vi "HH Cmd Interface.vi"(8 "error in":errorcluster, 9 "Device Inputs":dbl[](array[numeric]), 10 "DCM Ref":refnum<class "DCM - RT.lvclass">, 11 "HH in":T1) -> (0 "error out":errorcluster)   [LabVIEW 2016, in "DCM Engine.lvlib"]
uses:
  DCM Engine.lvlib
  Shared/Types/HH.ctl
  Shared/Types/HH Command Indexes.ctl
  Built/DCM Classes Packed/Pharlap/C/DCM-Classes.lvlibp/DCM/Rev0/RT/DCM - RT.lvclass
  Built/DCM Classes Packed/Pharlap/C/DCM-Classes.lvlibp/DCM/HH/RT/Setup.ctl
  Built/DCM Classes Packed/Pharlap/C/DCM-Classes.lvlibp/1abvi3w/vi.lib/Powertrain Controls/Device Drivers/DCM/HH/FPGA/Mode.ctl
  Built/DCM Classes Packed/Pharlap/C/DCM-Classes.lvlibp/1abvi3w/vi.lib/Powertrain Controls/Device Drivers/DCM/Rev0/FPGA/Digital Channel.ctl
  Built/DCM Classes Packed/Pharlap/C/DCM-Classes.lvlibp/DCM/HH/RT/Angle Control.ctl
  Built/DCM Classes Packed/Pharlap/C/DCM-Classes.lvlibp/DCM/HH/RT/DCM - RT - HH.lvlib
  Built/DCM Classes Packed/Pharlap/C/DCM-Classes.lvlibp/1abvi3w/vi.lib/Powertrain Controls/Device Drivers/DCM/HH/FPGA/DCM - FPGA - HH.lvlib
  Built/DCM Classes Packed/Pharlap/C/DCM-Classes.lvlibp/1abvi3w/vi.lib/Powertrain Controls/Device Drivers/DCM/Rev0/FPGA/DCM - FPGA.lvlib
  DCM Shared.lvlib
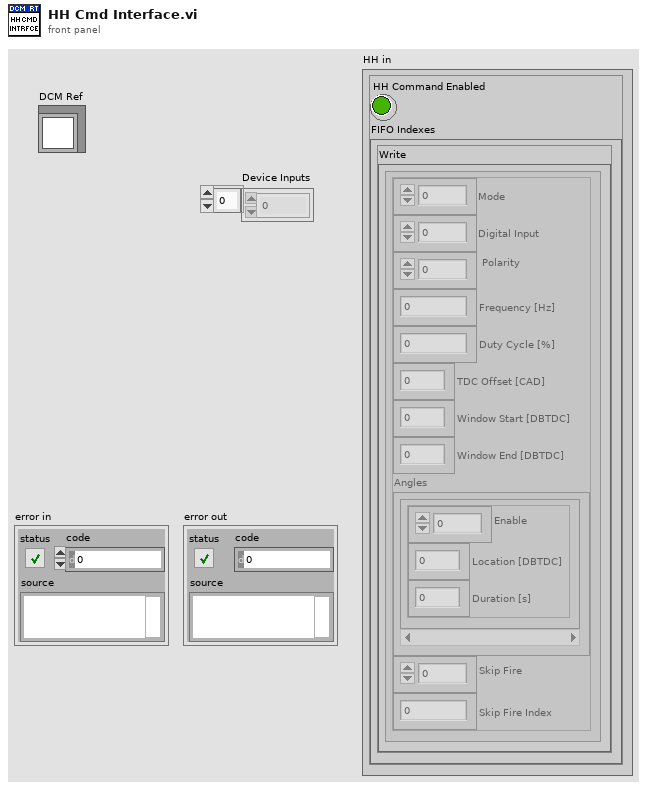
[diagram p1: front panel]
types:
  T1 = typedef "DCM Shared.lvlib/HH.ctl" = cluster{"HH Command Enabled":bool, "FIFO Indexes":cluster{"Write":T2[]}}
  T2 = typedef "DCM Shared.lvlib/HH Command Indexes.ctl" = cluster{"Mode":i32, "Digital Input":i32, "Polarity":i32, "Frequency [Hz]":i32, "Duty Cycle [%]":i32, "TDC Offset [CAD]":i32, "Window Start [DBTDC]":i32, "Window End [DBTDC]":i32, "Angles":cluster{"Enable":i32, "Location [DBTDC]":i32, "Duration [s]":i32}[], "Skip Fire":i32, "Skip Fire Index":i32}
  T3 = typedef "DCM-Classes.lvlibp/DCM - RT - HH.lvlib/Angle Control.ctl" = cluster{"Enable":bool, "Location [DBTDC]":sgl, "Duration [s]":sgl}
  T4 = typedef "DCM-Classes.lvlibp/DCM - RT - HH.lvlib/Setup.ctl" = cluster{"Mode":T5, "Digital Input":T6, "Polarity":bool, "Frequency [Hz]":sgl, "Duty Cycle [%]":sgl, "TDC Offset [CAD]":sgl, "Window Start [DBTDC]":sgl, "Window End [DBTDC]":sgl, "Angles":T3[], "Skip Fire":bool, "Skip Fire Index":u8}
  T5 = typedef "DCM-Classes.lvlibp/DCM - FPGA - HH.lvlib/Mode.ctl" = enum8{"Off", "Direct", "Pulse Width Modulation", "Engine Position Tracking"}
  T6 = typedef "DCM-Classes.lvlibp/DCM - FPGA.lvlib/Digital Channel.ctl" = enum8{"Unused", "User OS", "Diff IO 1", "Diff IO 2", "Diff IO 3", "Diff IO 4", "Diff IO 5", "Diff IO 6", "Diff IO 7", "Diff IO 8", "Aux 1", "Aux 2", "Aux 3", "Aux 4", "Aux 5", "Aux 6", "Aux 7", "Aux 8", "Aux 9", "Aux 10", "Aux 11", "Aux 12", "Aux 13", "Aux 14", "Aux 15", "Aux 16"}
  T7 = cluster{"Enable":i32, "Location [DBTDC]":i32, "Duration [s]":i32}[]
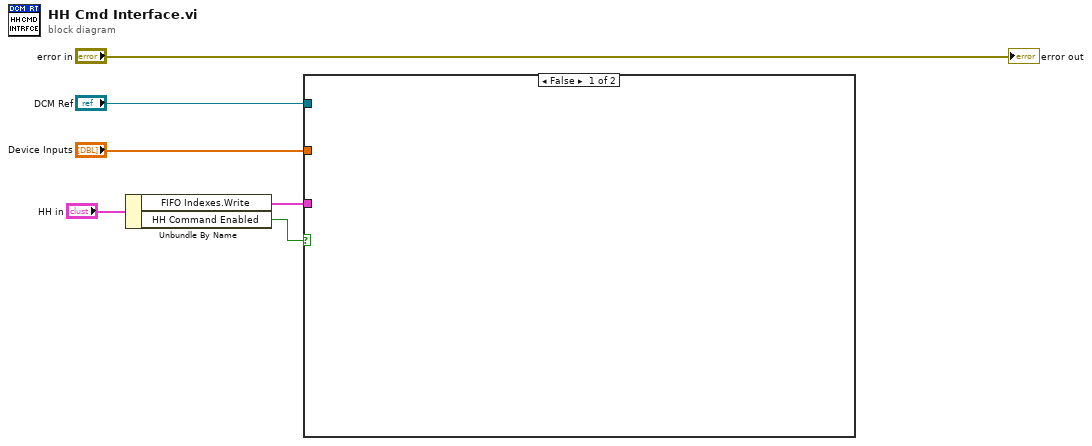
[diagram p0: block diagram]
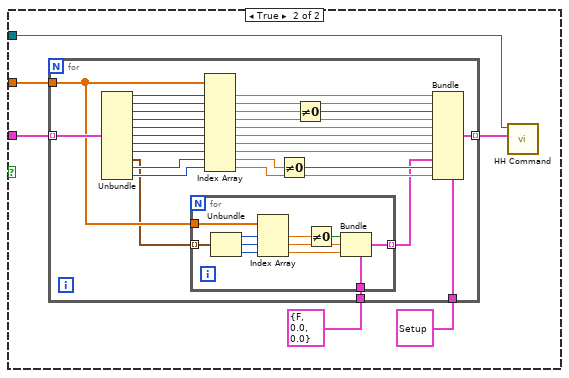
[diagram p2: hidden frame]
diagram:
  n1 = Unbundle By Name("HH in") -> ("FIFO Indexes.Write"=w3:T2[], "HH Command Enabled"=w2:bool)
  n2 = case shown="False" w2 {
    tunnel: "Device Inputs" -> [_ w12]
    tunnel: w3 -> [_ w11]
    tunnel: "DCM Ref" -> [_ w7]
    frame False {
    }
    frame True {
      n3 = for {
        tunnel: w12 -> [w16]
        tunnel: w11 -> [w41] mode=indexing
        tunnel: T3 {"Enable"=FALSE, "Location [DBTDC]"=0.0, "Duration [s]"=0.0} ("Injection Control") -> [w18]
        tunnel: T4 {"Mode"=enum."Off", "Digital Input"=enum."Unused", "Polarity"=FALSE, "Frequency [Hz]"=0.0, "Duty Cycle [%]"=0.0, "TDC Offset [CAD]"=0.0, "Window Start [DBTDC]"=0.0, "Window End [DBTDC]"=0.0, "Angles"=[{"Enable"=FALSE, "Location [DBTDC]"=0.0, "Duration [s]"=0.0}, {"Enable"=FALSE, "Location [DBTDC]"=0.0, "Duration [s]"=0.0}, {"Enable"=FALSE, "Location [DBTDC]"=0.0, "Duration [s]"=0.0}, {"Enable"=FALSE, "Location [DBTDC]"=0.0, "Duration [s]"=0.0}], "Skip Fire"=FALSE, "Skip Fire Index"=0} -> [w17]
        tunnel: [w13] -> w8 mode=indexing
        n4 = Unbundle(w41) -> ("Mode"=w40:i32, "Digital Input"=w39:i32, "Polarity"=w38:i32, "Frequency [Hz]"=w37:i32, "Duty Cycle [%]"=w36:i32, "TDC Offset [CAD]"=w35:i32, "Window Start [DBTDC]"=w34:i32, "Window End [DBTDC]"=w33:i32, "Angles"=w15:T7, "Skip Fire"=w32:i32, "Skip Fire Index"=w31:i32)
        n5 = for {
          tunnel: w18 -> [w52]
          tunnel: w16 -> [w51]
          tunnel: w15 -> [w50] mode=indexing
          tunnel: [w42] -> w14 mode=indexing
          n6 = Unbundle(w50) -> ("Enable"=w48:i32, "Location [DBTDC]"=w49:i32, "Duration [s]"=w47:i32)
          n7 = Index Array(array=w51, index #1=w48, index #2=w49, index #3=w47) -> (element #1=w46:dbl, element #2=w44:dbl, element #3=w43:dbl)
          n8 = Not Equal To 0?(x=w46) -> (x != 0?=w45:bool)
          n9 = Bundle(cluster=w52, "Enable"=w45, "Location [DBTDC]"=w44, "Duration [s]"=w43) -> (w42:T3)
        }
        n10 = Index Array(array=w16, index #1=w40, index #2=w39, index #3=w38, index #4=w37, index #5=w36, index #6=w35, index #7=w34, index #8=w33, index #9=w32, index #10=w31) -> (element #1=w30:dbl, element #2=w29:dbl, element #3=w28:dbl, element #4=w26:dbl, element #5=w24:dbl, element #6=w25:dbl, element #7=w23:dbl, element #8=w22:dbl, element #9=w20:dbl, element #10=w19:dbl)
        n11 = Not Equal To 0?(x=w20) -> (x != 0?=w21:bool)
        n12 = Not Equal To 0?(x=w28) -> (x != 0?=w27:bool)
        n13 = Bundle(cluster=w17, "Mode"=w30, "Digital Input"=w29, "Polarity"=w27, "Frequency [Hz]"=w26, "Duty Cycle [%]"=w24, "TDC Offset [CAD]"=w25, "Window Start [DBTDC]"=w23, "Window End [DBTDC]"=w22, "Angles"=w14, "Skip Fire"=w21, "Skip Fire Index"=w19) -> (w13:T4)
      }
      n14 = call "HH Command.vi"("HH Setup"=w8, "DCM Reference"=w7) -> ()  [unwired: 10 in]
    }
  }
  "error out" <- "error in"
